vi "Format Client Request (String).vi"(8 "error in (no error)":errorcluster, 9 "id":string, 10 "params":variant, 11 "method":string) -> (0 "error out":errorcluster, 2 "Request String":string)   [LabVIEW 2017, in "JSONRPC Client.lvclass"]
uses:
  JSONRPC Client.lvclass
  <vilib>/National Instruments/Variant Data Manipulation/Insert Element at Start.vi
  <vilib>/National Instruments/Variant Data Manipulation/Variant Data Manipulation.lvlib
  <vilib>/National Instruments/Variant JSON API/Variant JSON API.lvlib
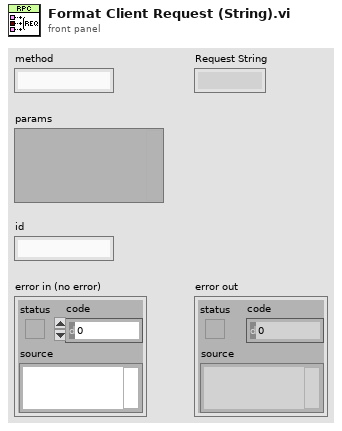
[diagram p1: front panel]
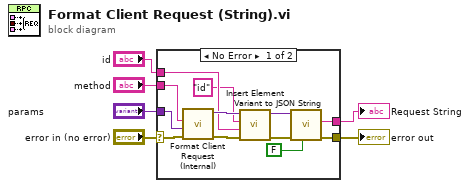
[diagram p0: block diagram]
diagram:
  n1 = case shown="No Error" "error in (no error)" {
    selector: "error in (no error)" -> [w18 w19]
    tunnel: [w17 w19] -> w5
    tunnel: "params" -> [w12 _]
    tunnel: [w16 _] -> w3
    tunnel: "method" -> [w15 _]
    tunnel: "id" -> [w8 _]
    frame No Error {
      n2 = call "Format Client Request (Internal).vi"("error in (no error)"=w18, "params"=w12, "method"=w15) -> ("error out"=w13:errorcluster, "JSON Value out"=w11:variant)  [unwired: 7 in]
      n3 = call-poly <vilib>:"Insert Element.vi"("error in (no error)"=w13, "element"=w8, "Name"="id", "Variant (Cluster) in"=w11) -> ("error out"=w14:errorcluster, "Variant (Cluster) out"=w10:variant)  [unwired: 6 in]
      n4 = call <vilib>:"Variant to JSON String.vi"("pretty print? (F)"=FALSE ("pretty print? (T)"), "error in (no error)"=w14, "Variant in"=w10) -> ("error out"=w17:errorcluster, "String"=w16:string)  [unwired: 6 in, 1 out]
    }
    frame Error {
    }
  }
  "error out" <- w5
  "Request String" <- w3
